vi "get limits.vi"(10 "4112?":bool=TRUE) -> (3 "output cluster":T1)   [LabVIEW 2023, in "NI PXIe-411x PS Custom Device.lvlib"]
uses:
  NI PXIe-411x PS Custom Device.lvlib
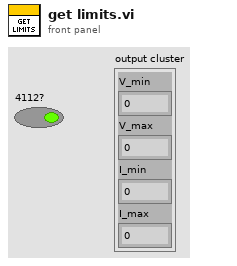
[diagram p1: front panel]
types:
  T1 = cluster{"V_min":dbl, "V_max":dbl, "I_min":dbl, "I_max":dbl}
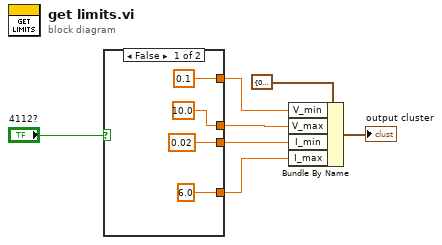
[diagram p0: block diagram]
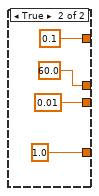
[diagram p2: hidden frame]
diagram:
  n1 = case shown="False" "4112?" {
    tunnel: [0.1 ("V_min") 0.1 ("V_min")] -> w3
    tunnel: [10.0 ("V_min") 60.0 ("V_min")] -> w4
    tunnel: [0.02 ("V_min") 0.01 ("V_min")] -> w5
    tunnel: [6.0 ("V_min") 1.0 ("t")] -> w6
    frame False {
    }
    frame True {
    }
  }
  n2 = Bundle By Name(cluster=T1 {"V_min"=0.0, "V_max"=0.0, "I_min"=0.0, "I_max"=0.0} ("output cluster"), "V_min"=w3, "V_max"=w4, "I_min"=w5, "I_max"=w6) -> (→"output cluster":T1)
